vi "create initialized module for testing.vi"() -> (0 "error out":errorcluster, 1 "2d channels":refnum<class "Profibus channel.lvclass">[][](array[class]), 2 "1d channels":refnum<class "Profibus channel.lvclass">[](array[class]), 3 "Profibus Module configuration out":refnum<class "Profibus Module configuration.lvclass">, 5 "2d names":string[][](array[string]), 7 "1d names":string[](array[string]))   [LabVIEW 2013, in "Profibus Module tests.lvlib"]
uses:
  Profibus Module tests.lvlib
  channel/Profibus channel.lvclass
  configuration/Profibus Module configuration.lvclass
  configuration/Profibus Module configuration.lvclass/Profibus Module configuration.ctl
  configuration/Write RIO interface.vi
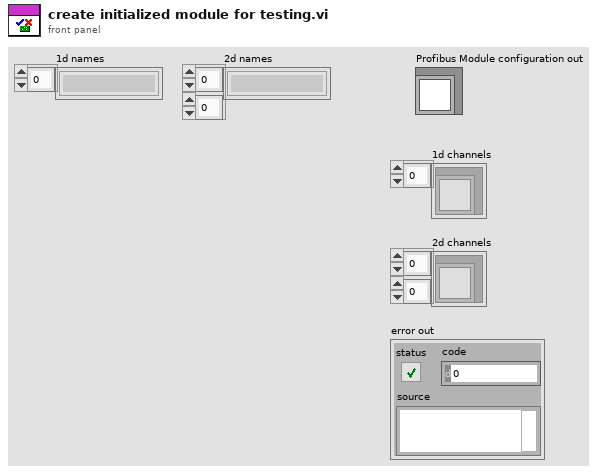
[diagram p1: front panel]
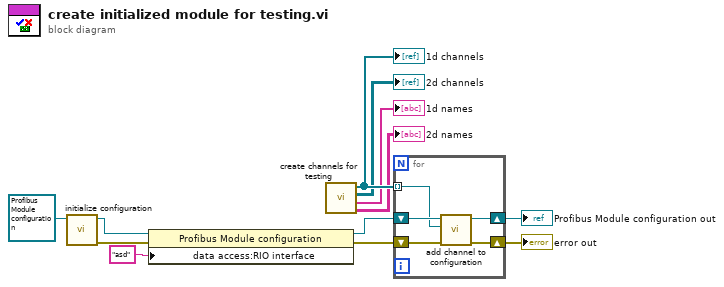
[diagram p0: block diagram]
diagram:
  n1 = call-dynamic "initialize configuration.vi"("configuration in"=refnum<class "Profibus Module configuration.lvclass"> refnum ("tag bus configurable plugin module configuration")) -> ("error out"=w11:errorcluster, "configuration out"=w3:refnum<class "Profibus Module configuration.lvclass">)  [unwired: 8 in, 1 out]
  n2 = property class="Profibus Module configuration"(reference=w3, error in=w11, "data access:RIO interface"="asd" ("RIO interface")) -> (reference out=w2:refnum<class "Profibus Module configuration.lvclass">, error out=w4:errorcluster)
  n3 = call "create channels for testing.vi"() -> ("2d names"=→"2d names":string[][], "1d names"=→"1d names":string[], "2d channels"=→"2d channels":refnum<class "Profibus channel.lvclass">[][], "1d channels"=w12:refnum<class "Profibus channel.lvclass">[])  [unwired: 8 in]
  "1d channels" <- w12
  n4 = for {
    tunnel: w12 -> [w15] mode=indexing
    shift-right: [w14] -> w8
    shift-left: w2 -> [w17]
    shift-right: [w13] -> w9
    shift-left: w4 -> [w16]
    n5 = call "add channel to configuration.vi"("error in"=w16, "TBM channel in"=w15, "Profibus Module configuration in"=w17) -> ("error out"=w13:errorcluster, "Profibus Module configuration out"=w14:refnum<class "Profibus Module configuration.lvclass">)  [unwired: 7 in]
  }
  "error out" <- w9
  "Profibus Module configuration out" <- w8
